vi "Unpack Notification Msg.vi"(11 "Notification Msg":refnum<class "Notification Msg.lvclass">) -> (1 "Publication Time":timestamp, 2 "Value":variant, 3 "Datum Name":string)   [LabVIEW 2020, in "ActorMessageTransport.lvlib" / "Notification Msg.lvclass"]
doc: "从已完成的通知消息中解压缩数据。\n***不要覆盖此方法***\n此方法中添加了动态调度，以实现MVA框架中的向后兼容性。DD将在未来的版本中删除。"
uses:
  Notification Msg.lvclass
  Notification Msg.lvclass/Notification Msg.ctl
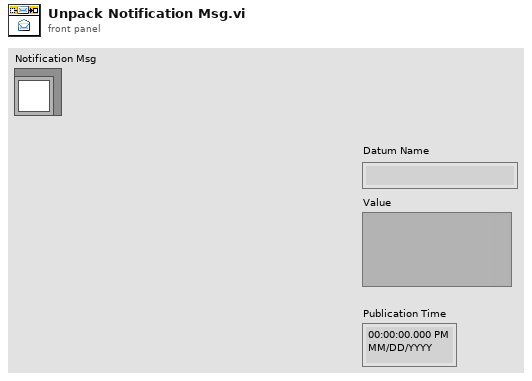
[diagram p1: front panel]
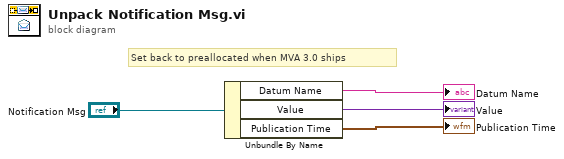
[diagram p0: block diagram]
diagram:
  # "Set back to preallocated when MVA 3.0 ships"
  n1 = Unbundle By Name("Notification Msg") -> ("Datum Name"=→"Datum Name":string, "Value"=→"Value":variant, "Publication Time"=→"Publication Time":timestamp)
